vi "Stability.vi"(0 "Stability Parameters":T2={"Window 1 time (s)"=2e-05, "Window 2 time (s)"=1e-06, "Window 3 time (s) "=5e-08, "Window 4 time (s)"=2e-06, "Window 5 time (s)"=1e-07, "Window 6 time (s)"=5e-08, "Path to StabilityBurn"=path "C:/Users/Loncar/Desktop/ESR VIs - Srujan/Sam Kim/PB/StabilityBurn.exe", "Window 1 active channels"=[FALSE, TRUE], "Window 2 active channels"=[], "Window 3 active channels "=[FALSE, FALSE, TRUE], "Window 4 active channels"=[TRUE, FALSE, TRUE], "Window 5 active channels"=[FALSE, FALSE, TRUE], "Window 6 active channels"=[]}, 1 "Optimize Parameters":T1={"Volt Step"={"X"=0.01, "Y"=0.01, "Z"=0.0}, "Num Iterations"=1, "Dwell Time (ms)"=100, "Volts Range"={"X"=0.1, "Y"=0.1, "Z"=0.0}, "Method"={"X"=enum."Max", "Y"=enum."Max"}} {"Volts Range"."Z" min=0.0; "Volts Range"."Y" min=0.0; "Volts Range"."X" min=0.0; "Dwell Time (ms)" min=0; "Num Iterations" min=1 step=1; "Volt Step"."Z" min=0.0; "Volt Step"."Y" min=1e-06; "Volt Step"."X" min=1e-06}, 2 "# Scans":i32, 3 "V min":dbl=-0.3, 4 "V max":dbl=0.3, 5 "# V steps":dbl, 6 "Save 2D counts array to spreadsheet":bool, 7 "Num Scan Iterations":i32, 8 "Path for 2D counts spreadsheet":path=path "C:/experiment/data/may_15_2012/SIL1_NV1_pippin_uW_off", 9 "Counts vs laser IntGraph Refnum":refnum<vi>, 10 "Save intensity graph":bool, 11 "Pict Refnum":refnum<vi>, 12 "Path for intensity graph":path=path "C:/experiment/data/may_15_2012/SIL1_NV1_pippin_uW_off", 14 "Save avg counts data":bool, 15 "Path for avg spectrum spreadsheet":path=path "C:/experiment/data/may_15_2012/SIL1_NV1_pippin_uW_off", 16 "Save avg spectrum graph?":bool, 17 "Path for avg spectrum graph":path=path "C:/experiment/data/may_15_2012/SIL1_NV1_pippin_uW_off") -> ()   [LabVIEW 2012]
uses:
  <vilib>/Analysis/NI_AALBase.lvlib
  <vilib>/Analysis/baseanly.llb/Mean (DBL).vi
  <vilib>/Utility/file.llb/Write To Spreadsheet File (DBL).vi
  <vilib>/DAQmx/read.llb/DAQmx Read (Counter 1D U32 1Chan NSamp).vi
  Channels.vi
  Global Vars.vi
  Stability Window Parameters.ctl
  Strict Type Def - Optimize Parameters Cluster.ctl
panel:
  out "Average counts":picture
  out "Counts vs. laser voltage":u32[][](graph)
  out "2D array of # counts":u32[][](array[numeric])
  # "VI for spectral stability characterization\nDated: 05/27/2013\nCorrection 1: 08/05/2013\nCorrection 2: 08/26/2013"
  # "Default PB connections:\nPB0 - Red AOM\nPB1 - Green AOM\nPB2 - Counter sample clk"
  # "Window descriptions and states of PB signals:\n1. Green AOM on\n2. All off\n3. Counter sample clk on\n4. Red AOM on, counter sample clk on\n5. Counter sample clk on\n6. All off\n\nConsidering AOM delay, try making the foll changes:\n1. Green AOM on - few us (take turn-on time into consideration)\n2. Red AOM on - 0.75 us (during this window, green AOM turns off and red AOM turns on)\n3. Red AOM on, counter sample clk on - custom\n4. Counter sample clk on - 0.75 us (during this period red AOM turns off)"
  # "Laser Set:"
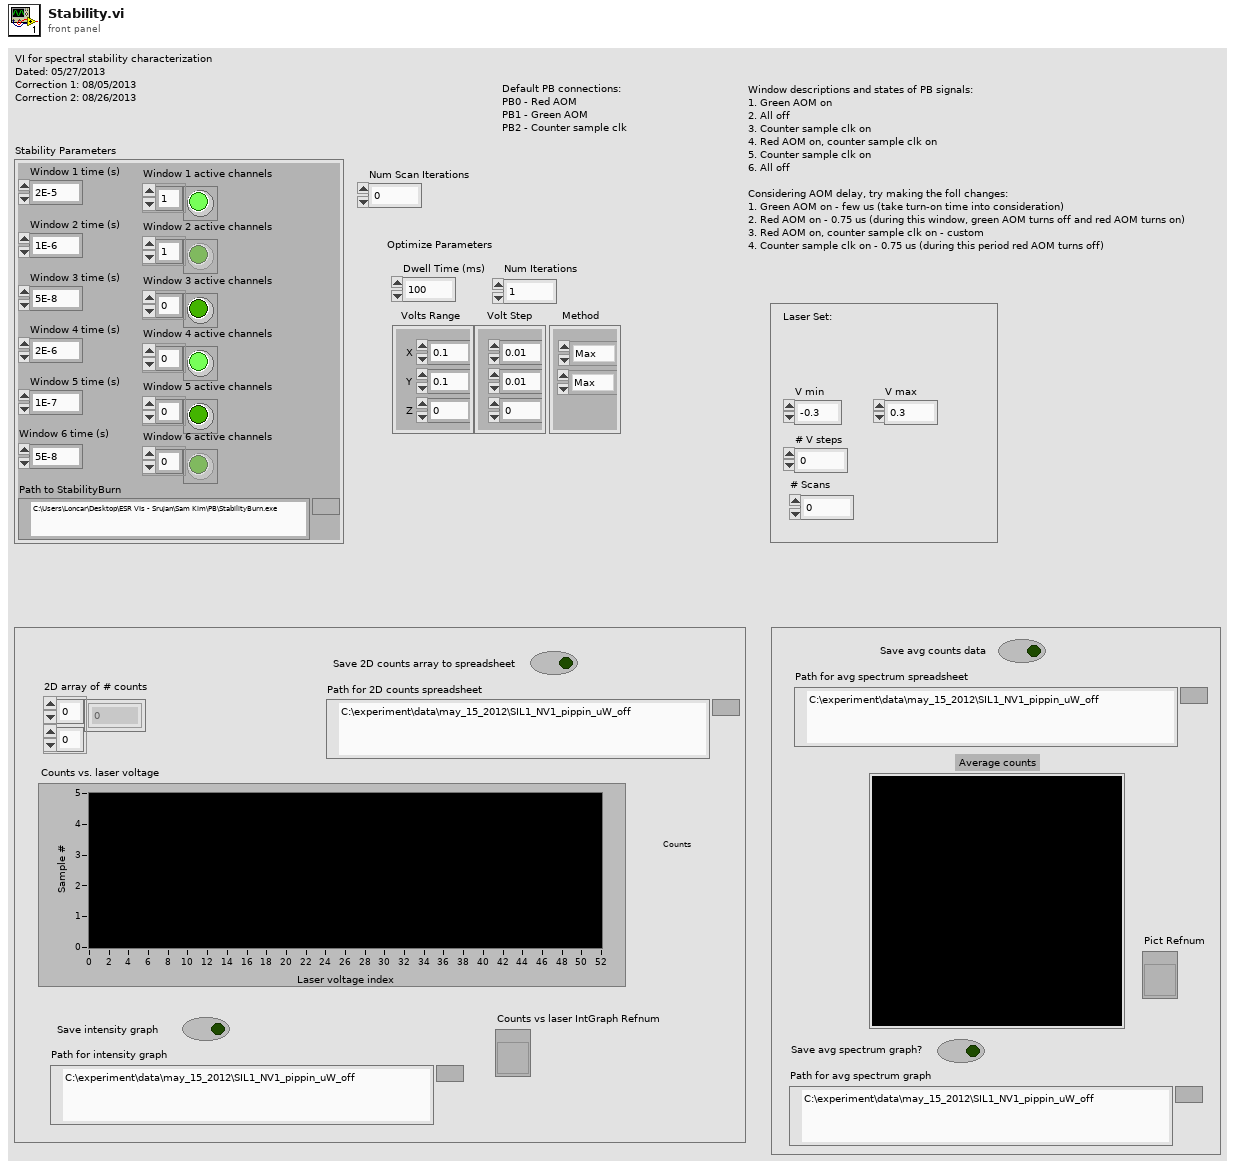
[diagram p1: front panel]
types:
  T1 = typedef "Strict Type Def - Optimize Parameters Cluster.ctl" = cluster{"Volt Step":cluster{"X":dbl, "Y":dbl, "Z":dbl}, "Num Iterations":i32, "Dwell Time (ms)":i32, "Volts Range":cluster{"X":dbl, "Y":dbl, "Z":dbl}, "Method":cluster{"X":enum16{"Max", "Gaussian"}, "Y":enum16{"Max", "Gaussian"}}}
  T2 = typedef "Stability Window Parameters.ctl" = cluster{"Window 1 time (s)":dbl, "Window 2 time (s)":dbl, "Window 3 time (s) ":dbl, "Window 4 time (s)":dbl, "Window 5 time (s)":dbl, "Window 6 time (s)":dbl, "Path to StabilityBurn":path, "Window 1 active channels":bool[], "Window 2 active channels":bool[], "Window 3 active channels ":bool[], "Window 4 active channels":bool[], "Window 5 active channels":bool[], "Window 6 active channels":bool[]}
  T3 = typedef "imagedata.ctl" = cluster{"image type":i32, "image depth":i32, "image":u8[], "mask":u8[], "colors":u32[], "Rectangle":cluster{"left":i16, "top":i16, "right":i16, "bottom":i16}}
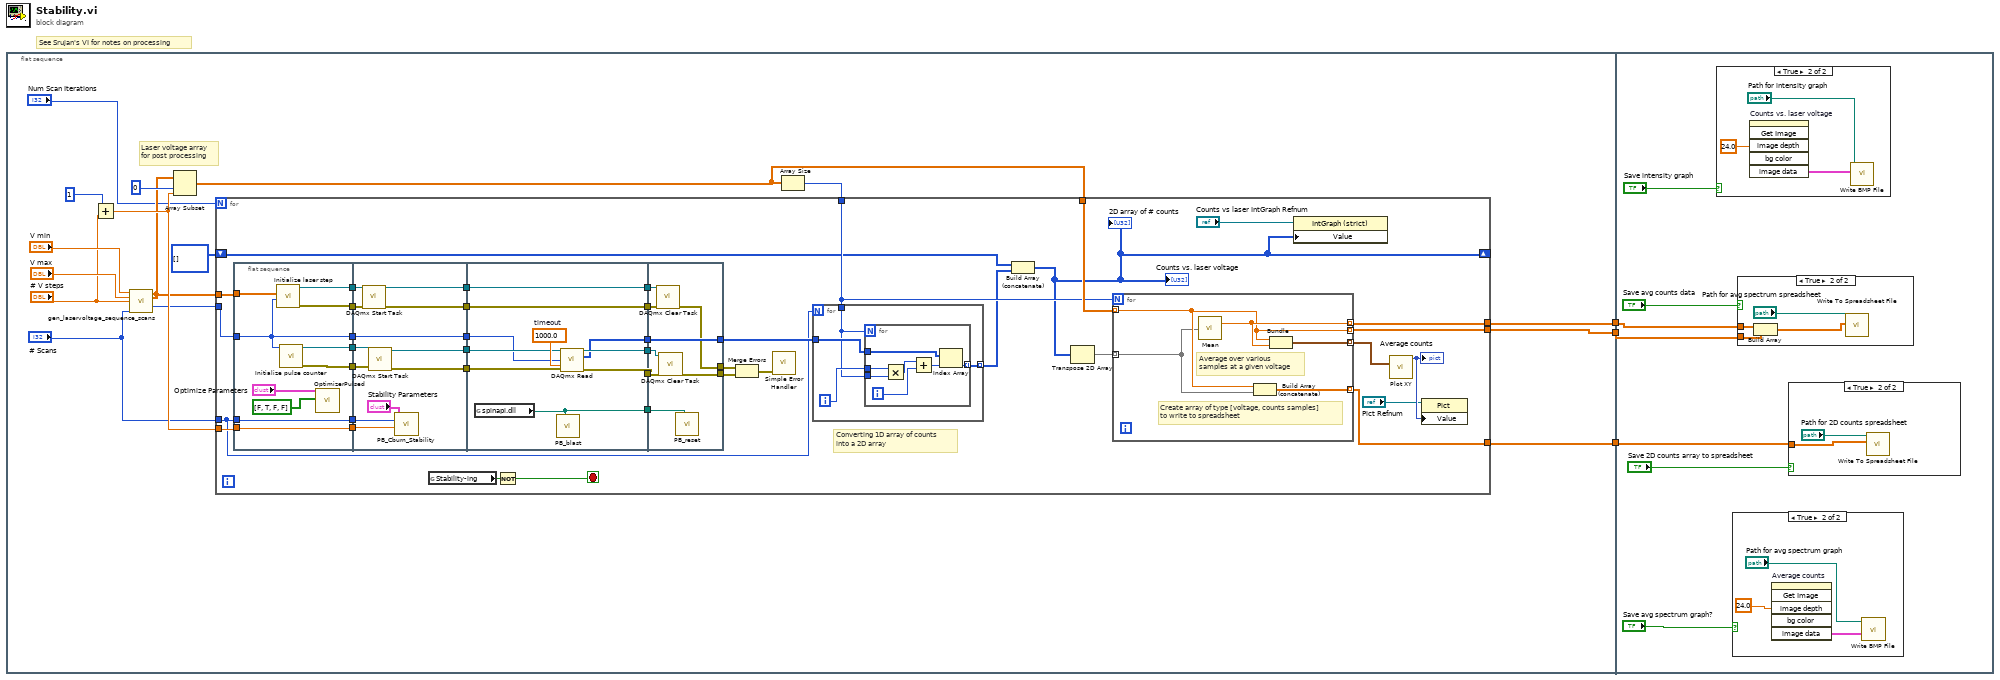
[diagram p0: block diagram]
diagram:
  # "See Srujan's VI for notes on processing"
  n1 = flat-sequence {
    tunnel: [w19] -> w3
    tunnel: [w18] -> w2
    tunnel: [w17] -> w1
    tunnel: w3 -> [w120]
    tunnel: w2 -> [w119]
    tunnel: w1 -> [w117]
    frame #0 {
      # "Laser voltage array\nfor post processing"
      n2 = Add(x=u32 1 ("Reset Count"), y="# V steps") -> (x+y=w10:dbl)
      n3 = call "gen_laservoltage_sequence_scans.vi"("V min"="V min", "V max"="V max", "# V steps"="# V steps", "# Scans"="# Scans") -> ("Voltage sequence"=w7:dbl[], "Total # data points"=w6:i32)  [unwired: 10 in]
      n4 = Array Subset(array=w7, index=u32 0 ("Reset Count"), length=w10) -> (w12:dbl[])
      n5 = Array Size(array=w12) -> (size(s)=w8:i32)
      n6 = for {
        N: "Num Scan Iterations" -> [_]
        tunnel: [w41] -> w19
        tunnel: [w40] -> w18
        tunnel: [w39] -> w17
        tunnel: w12 -> [w35]
        tunnel: w10 -> [w34]
        tunnel: "# Scans" -> [w33]
        tunnel: w8 -> [w32]
        tunnel: w7 -> [w29]
        tunnel: w6 -> [w28]
        shift-right: [w22] -> _
        shift-left: i32[][] [] ("Flourescence Data") -> [w27]
        stop <- w24 stop-if-true
        # "Converting 1D array of counts \ninto a 2D array"
        n7 = flat-sequence {
          tunnel: w33 -> [w80]
          tunnel: w34 -> [w81]
          tunnel: w28 -> [w74]
          tunnel: [w76] -> w60
          tunnel: [w75] -> w59
          tunnel: [w74] -> w58
          tunnel: [w79] -> w57
          tunnel: [w78] -> w56
          tunnel: [w81] -> w55
          tunnel: [w80] -> w54
          tunnel: w29 -> [w77]
          tunnel: [w91] -> w53
          tunnel: [w90] -> w52
          tunnel: [w87] -> w51
          tunnel: [w86] -> w50
          tunnel: [w85] -> w49
          tunnel: w60 -> [w93]
          tunnel: w59 -> [w92]
          tunnel: w58 -> [w85]
          tunnel: w57 -> [w89]
          tunnel: w56 -> [w88]
          tunnel: w55 -> [w83]
          tunnel: w54 -> [w84]
          tunnel: w53 -> [w102]
          tunnel: w52 -> [w101]
          tunnel: [w96] -> w48
          tunnel: [w100] -> w47
          tunnel: [w99] -> w46
          tunnel: [w98] -> w45
          tunnel: w51 -> [w98]
          tunnel: w50 -> [w97]
          tunnel: [w97] -> w44
          tunnel: w49 -> [w95]
          tunnel: [w94] -> w43
          tunnel: [w111] -> w36
          tunnel: w48 -> [w111]
          tunnel: w47 -> [w110]
          tunnel: w46 -> [w109]
          tunnel: w45 -> [w106]
          tunnel: w44 -> [w105]
          tunnel: [w108] -> w38
          tunnel: w43 -> [w107]
          tunnel: [w104] -> w30
          frame #0 {
            n8 = call "Initialize laser step.vi"("Total # data points"=w74, "Voltage sequence"=w77) -> ("error out"=w78:errorcluster, "Task out"=w79:refnum<k21>)  [unwired: 8 in]
            n9 = call "Initialize pulse counter.vi"("Samples per channel"=w74) -> ("error out"=w75:errorcluster, "DAQmx Task Name"=w76:refnum<k21>)  [unwired: 9 in]
            n10 = call "OptimizerPulsed.vi"("Optimize active channels"=bool[] [FALSE, TRUE, FALSE, FALSE], "Optimize Parameters"="Optimize Parameters") -> ()  [unwired: 9 in, 1 out]
          }
          frame #1 {
            n11 = call <vilib>:"DAQmx Start Task.vi"("task/channels in"=w89, "error in"=w88) -> ("task out"=w87:refnum<k21>, "error out"=w86:errorcluster)  [unwired: 12 in]
            n12 = call <vilib>:"DAQmx Start Task.vi"("task/channels in"=w93, "error in"=w92) -> ("task out"=w91:refnum<k21>, "error out"=w90:errorcluster)  [unwired: 12 in]
            n13 = call "PB_Cburn_Stability.vi"("Spectrum Parameters"="Stability Parameters", "# scans before track"=w84, "# steps"=w83) -> ()  [unwired: 7 in, 1 out]
          }
          frame #2 {
            w103 = 1000.0  # timeout
            n14 = global read "Channels.vi" "spinapi.dll"() -> (w94:path)
            n15 = call "PB_blast.vi"("Path to spinapi.dll"=w94) -> ()  [unwired: 7 in]
            n16 = call-poly <vilib>:"DAQmx Read.vi"("task/channels in"=w102, "number of samples per channel"=w95, "timeout"=w103, "error in"=w101) -> ("task out"=w99:refnum<k21>, "data"=w96:u32[], "error out"=w100:errorcluster)  [unwired: 9 in]
          }
          frame #3 {
            n17 = call <vilib>:"DAQmx Clear Task.vi"("task in"=w106, "error in"=w105) -> ("error out"=w104:errorcluster)  [unwired: 13 in]
            n18 = call <vilib>:"DAQmx Clear Task.vi"("task in"=w109, "error in"=w110) -> ("error out"=w108:errorcluster)  [unwired: 13 in]
            n19 = call "PB_reset.vi"("Path to spinapi.dll"=w107) -> ()  [unwired: 7 in]
          }
        }
        n20 = global read "Global Vars.vi" "Stability-ing"() -> (w25:bool)
        n21 = Not(x=w25) -> (.not. x?=w24:bool)
        n22 = Merge Errors(w30, w38) -> (w37:errorcluster)
        n23 = call <vilib>:"Simple Error Handler.vi"("error in (no error)"=w37) -> ()  [unwired: 4 in, 5 out]
        n24 = for {
          N: w33 -> [_]
          tunnel: w36 -> [w64]
          tunnel: w32 -> [w61]
          tunnel: [w63] -> w26 mode=indexing
          i -> [w62]
          n25 = for {
            N: w61 -> [_]
            tunnel: w62 -> [w71]
            tunnel: w64 -> [w69]
            tunnel: [w68] -> w63 mode=indexing
            tunnel: w61 -> [w66]
            i -> [w67]
            n26 = Multiply(x=w71, y=w66) -> (x*y=w65:i32)
            n27 = Add(x=w65, y=w67) -> (x+y=w70:i32)
            n28 = Index Array(array=w69, index=w70) -> (element=w68:u32)
          }
        }
        n29 = Build Array (concatenate)(w27, w26) -> (w22:u32[][])
        "2D array of # counts" <- w22
        "Counts vs. laser voltage" <- w22
        n30 = Transpose 2D Array(2D array=w22) -> (transposed array=w31:u32[][])
        n31 = for {
          N: w32 -> [_]
          tunnel: [w116] -> w42 mode=indexing
          tunnel: [w113] -> w41 mode=indexing
          tunnel: [w115] -> w40 mode=indexing
          tunnel: [w114] -> w39 mode=indexing
          tunnel: w35 -> [w113] mode=indexing
          tunnel: w31 -> [w112] mode=indexing
          # "Create array of type [voltage, counts samples]\nto write to spreadsheet"
          # "Average over various \nsamples at a given voltage"
          n32 = call-poly <vilib>:"Mean.vi"("X"=w112) -> ("mean"=w115:dbl)  [unwired: 1 out]
          n33 = Build Array (concatenate)(w113, w112) -> (w114:dbl[])
          n34 = Bundle("element"=w113, "mean"=w115) -> (w116:cluster{"element":dbl, "mean":dbl})  [unwired: 1 in]
        }
        n35 = property class="IntGraph (strict)"(reference="Counts vs laser IntGraph Refnum", "Value"=w22) -> ()  [unwired: 1 in, 2 out]
        n36 = call <vilib>:"Plot XY.vi"("data"=w42) -> ("new picture"=w21:picture)  [unwired: 14 in]
        "Average counts" <- w21
        n37 = property class="Pict"(reference="Pict Refnum", "Value"=w21) -> ()  [unwired: 1 in, 2 out]
      }
    }
    frame #1 {
      n38 = case shown="True" "Save intensity graph" {
        frame False {
        }
        frame True {
          n39 = invoke on="Counts vs. laser voltage" class="IntGraph (strict)" method="Get Image"("image depth"=24.0 ("Initial Delay")) -> ("image data"=w135:T3)  [unwired: 5 in, 5 out]
          n40 = call <vilib>:"Write BMP File.vi"("image data"=w135, "path to BMP file"="Path for intensity graph") -> ()  [unwired: 8 in, 2 out]
        }
      }
      n41 = case shown="True" "Save avg spectrum graph?" {
        frame False {
        }
        frame True {
          n42 = invoke on="Average counts" class="Pict" method="Get Image"("image depth"=24.0 ("Initial Delay")) -> ("image data"=w131:T3)  [unwired: 5 in, 5 out]
          n43 = call <vilib>:"Write BMP File.vi"("image data"=w131, "path to BMP file"="Path for avg spectrum graph") -> ()  [unwired: 8 in, 2 out]
        }
      }
      n44 = case shown="True" "Save avg counts data" {
        tunnel: w120 -> [_ w127]
        tunnel: w119 -> [_ w128]
        frame False {
        }
        frame True {
          n45 = Build Array(w128, w127) -> (w126:dbl[][])
          n46 = call-poly <vilib>:"Write To Spreadsheet File.vi"("2D data"=w126, "file path (dialog if empty)"="Path for avg spectrum spreadsheet") -> ()  [unwired: 6 in, 1 out]
        }
      }
      n47 = case shown="True" "Save 2D counts array to spreadsheet" {
        tunnel: w117 -> [_ w124]
        frame False {
        }
        frame True {
          n48 = call-poly <vilib>:"Write To Spreadsheet File.vi"("2D data"=w124, "file path (dialog if empty)"="Path for 2D counts spreadsheet") -> ()  [unwired: 6 in, 1 out]
        }
      }
    }
  }
